vi "PSTR-Show Summary.vi"(0 "Data":T1, 5 "XYGraph":refnum<vi>) -> ()   [LabVIEW 2020]
uses:
  Typedefs/PSTR-Data.ctl
  Typedefs/PSTR-Model Fit.ctl
  Typedefs/PSTR-Fit Parameters.ctl
panel:
  # "NF x NL x 2 x Npts"
  # "NF x NL x Npts"
  # "NF x NL"
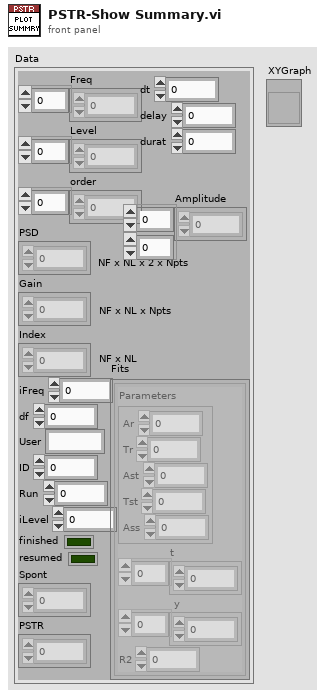
[diagram p1: front panel]
types:
  T1 = typedef "PSTR-Data.ctl" = cluster{"Freq":dbl[], "Level":dbl[], "order":i32[], "PSD":dbl[][][][], "Gain":dbl[][][], "Index":dbl[][], "iFreq":i32, "df":dbl, "User":string, "ID":i32, "Run":i32, "iLevel":i32, "finished":bool, "resumed":bool, "Spont":dbl[][], "PSTR":dbl[][][], "dt":dbl, "delay":dbl, "durat":dbl, "Fits":T2[][], "Amplitude":dbl[][]}
  T2 = typedef "PSTR-Model Fit.ctl" = cluster{"Parameters":T3, "t":dbl[], "y":dbl[], "R2":dbl}
  T3 = typedef "PSTR-Fit Parameters.ctl" = cluster{"Ar":dbl, "Tr":dbl, "Ast":dbl, "Tst":dbl, "Ass":dbl}
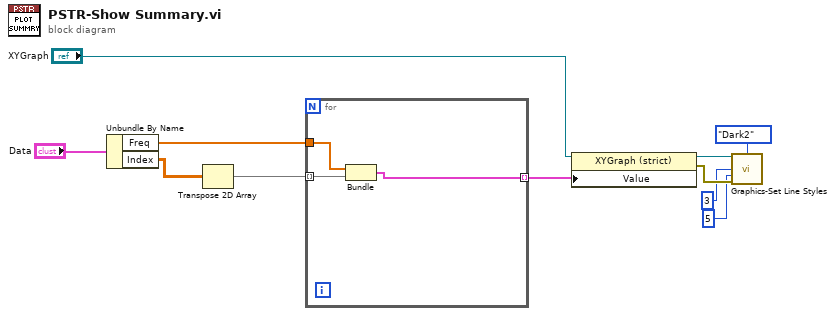
[diagram p0: block diagram]
diagram:
  n1 = Unbundle By Name("Data") -> ("Freq"=w7:dbl[], "Index"=w10:dbl[][])
  n2 = Transpose 2D Array(2D array=w10) -> (transposed array=w6:dbl[][])
  n3 = for {
    tunnel: w6 -> [w14] mode=indexing
    tunnel: [w12] -> w9 mode=indexing
    tunnel: w7 -> [w13]
    n4 = Bundle("Freq"=w13, w14) -> (w12:cluster{"Freq":dbl[], dbl[]})  [unwired: 1 in]
  }
  n5 = property class="XYGraph (strict)"(reference="XYGraph", "Value"=w9) -> (reference out=w5:refnum<vi>, error out=w4:errorcluster)  [unwired: 1 in]
  n6 = call "Graphics-Set Line Styles.vi"("XY Graph"=w5, "Map"=enum16{"User", "Prism", "Kelly", "Dark2"}."Dark2", "Plot.Line Width"=u8 3, "Plot.Point Style"=u8 5, "error in (no error)"=w4) -> ()  [unwired: 9 in, 2 out]
